vi "GripSensorConversion_r2.vi"(1 "Grip Sensor Output (g)":dbl) -> (0 "Grip Force (N)":dbl)   [LabVIEW 2020]
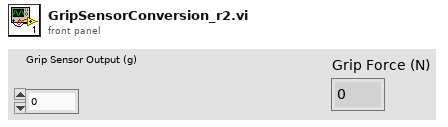
[diagram p1: front panel]
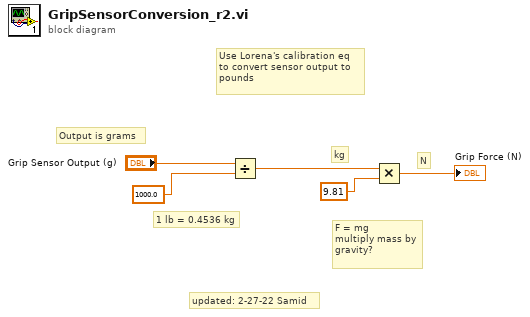
[diagram p0: block diagram]
diagram:
  # "updated: 2-27-22 Samid"
  # "N"
  # "kg"
  # "1 lb = 0.4536 kg"
  # "Use Lorena's calibration eq\nto convert sensor output to\npounds"
  # "Output is grams"
  # "F = mg\nmultiply mass by gravity?"
  n1 = Divide(x="Grip Sensor Output (g)", y=1000.0 ("x")) -> (x/y=w1:dbl)
  n2 = Multiply(x=w1, y=9.81 ("x")) -> (x*y=→"Grip Force (N)":dbl)
